vi "Database.Main-WriteValues.vi"(8 "error in":errorcluster, 10 "FileName":string) -> (0 "error out":errorcluster, 2 "Saved":bool)   [LabVIEW 2016]
doc: "Go to DB->WriteStationValues action\nReturn boolean flag to show if data was saved to DB successfully\n\nWabco 2017 All right reserved\nAuthor: maciej.szupienko@wabco-auto.com"
uses:
  Database.Main.Action.ctl
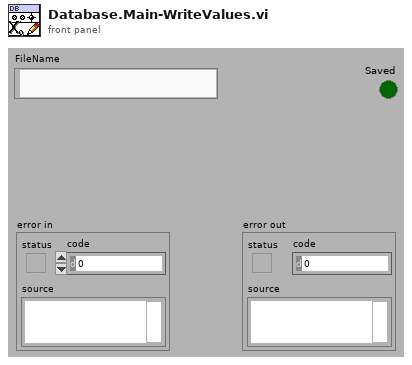
[diagram p1: front panel]
types:
  T1 = typedef "Database.Main.Action.ctl" = enum32{"idle", "constructor", "destructor", "--- DB ---", "Init", "Setup", "Select.Variant", "WriteValues"}
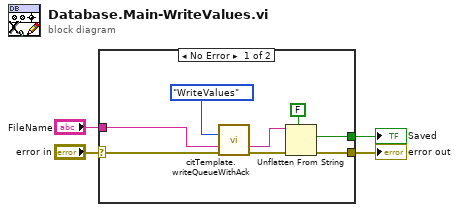
[diagram p0: block diagram]
diagram:
  n1 = case shown="No Error" "error in" {
    selector: "error in" -> [w5 w13]
    tunnel: [w11 w13] -> w3
    tunnel: [w7 _] -> w2
    tunnel: "FileName" -> [w6 _]
    frame No Error {
      n2 = call "citTemplate.writeQueueWithAck.vi"("event in"=Database.Main.Action."WriteValues" ("Action"), "(flatten) data in"=w6, "error in (no error)"=w5) -> ("notification data"=w10:string, "error out"=w12:errorcluster)  [unwired: 10 in, 1 out]
      n3 = Unflatten From String(type=FALSE, binary string=w10, error in (no error)=w12) -> (value=w7:bool, error out=w11:errorcluster)  [unwired: 2 in, 1 out]
    }
    frame Error {
    }
  }
  "error out" <- w3
  "Saved" <- w2
